vi "0 to N sum.vi"() -> ()   [LabVIEW 2010]
panel:
  in  "Numeric 3":dbl
  in  "Numeric 4":i8
  out "Numeric 2":i32
  in  "N value":i32=3
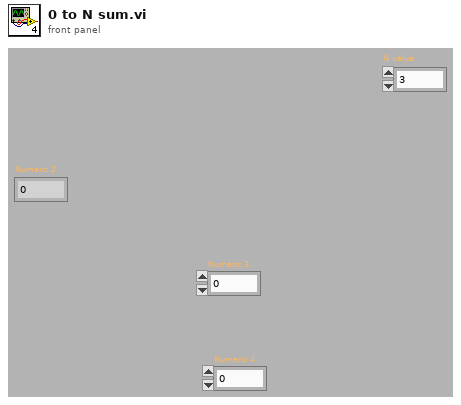
[diagram p1: front panel]
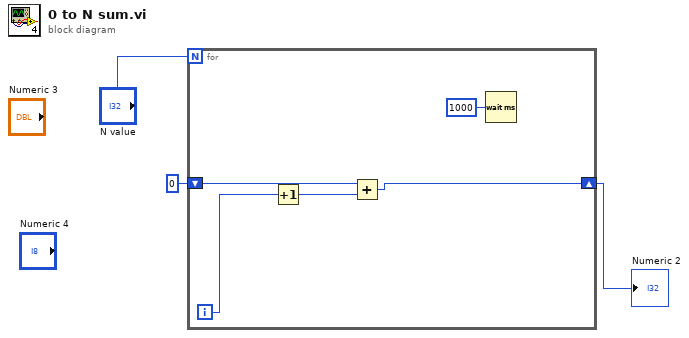
[diagram p0: block diagram]
diagram:
  n1 = for {
    N: "N value" -> [_]
    shift-right: [w5] -> w2
    shift-left: 0 -> [w4]
    i -> [w7]
    n2 = Increment(x=w7) -> (x+1=w6:i32)
    n3 = Add(x=w4, y=w6) -> (x+y=w5:i32)
    n4 = Wait (ms)(milliseconds to wait=u32 1000) -> ()  [unwired: 1 out]
  }
  "Numeric 2" <- w2
